vi "PicohrdlChannelSetting.vi"(5 "Unit Info":T1, 7 "Channel Settings":T2={"Ch1"={"1"=FALSE, "Ch 1"=0}, "Ch2"={"2"=FALSE, "Ch 2"=0}, "Ch3"={"3"=FALSE, "Ch 3"=0}, "Ch4"={"4"=FALSE, "Ch 4"=0}, "Ch5"={"5"=FALSE, "Ch 5"=0}, "Ch6"={"6"=FALSE, "Ch 6"=0}, "Ch7"={"7"=FALSE, "Ch 7"=0}, "Ch8"={"8"=FALSE, "Ch 8"=0}, "Ch9"={"9"=FALSE, "Ch 9"=0}, "Ch10"={"10"=FALSE, "Ch 10"=0}, "Ch11"={"11"=FALSE, "Ch 11"=0}, "Ch12"={"12"=FALSE, "Ch 12"=0}, "Ch13"={"13"=FALSE, "Ch 13"=0}, "Ch14"={"14"=FALSE, "Ch 14"=0}, "Ch15"={"15"=FALSE, "Ch 15"=0}, "Ch16"={"16"=FALSE, "Ch 16"=0}, "Ch1/Ch2"={"Single Ended"=TRUE}, "Ch3/Ch4"={"Single Ended"=TRUE}, "Ch5/Ch6"={"Single Ended"=TRUE}, "Ch7/Ch8"={"Single Ended"=TRUE}, "Ch9/Ch10"={"Single Ended"=TRUE}, "Ch11/Ch12"={"Single Ended"=TRUE}, "Ch13/Ch14"={"Single Ended"=TRUE}, "Ch15/Ch16"={"Single Ended"=TRUE}} {"Ch16"."Ch 16" items=["2500mV", "1225mV", "625mV", "313mV", "156mV", "78mV", "39mV"]; "Ch15"."Ch 15" items=["2500mV", "1225mV", "625mV", "313mV", "156mV", "78mV", "39mV"]; "Ch14"."Ch 14" items=["2500mV", "1225mV", "625mV", "313mV", "156mV", "78mV", "39mV"]; "Ch13"."Ch 13" items=["2500mV", "1225mV", "625mV", "313mV", "156mV", "78mV", "39mV"]; "Ch12"."Ch 12" items=["2500mV", "1225mV", "625mV", "313mV", "156mV", "78mV", "39mV"]; "Ch11"."Ch 11" items=["2500mV", "1225mV", "625mV", "313mV", "156mV", "78mV", "39mV"]; "Ch10"."Ch 10" items=["2500mV", "1225mV", "625mV", "313mV", "156mV", "78mV", "39mV"]; "Ch9"."Ch 9" items=["2500mV", "1225mV", "625mV", "313mV", "156mV", "78mV", "39mV"]; "Ch8"."Ch 8" items=["2500mV", "1225mV", "625mV", "313mV", "156mV", "78mV", "39mV"]; "Ch7"."Ch 7" items=["2500mV", "1225mV", "625mV", "313mV", "156mV", "78mV", "39mV"]; "Ch6"."Ch 6" items=["2500mV", "1225mV", "625mV", "313mV", "156mV", "78mV", "39mV"]; "Ch5"."Ch 5" items=["2500mV", "1225mV", "625mV", "313mV", "156mV", "78mV", "39mV"]; "Ch4"."Ch 4" items=["2500mV", "1225mV", "625mV", "313mV", "156mV", "78mV", "39mV"]; "Ch3"."Ch 3" items=["2500mV", "1225mV", "625mV", "313mV", "156mV", "78mV", "39mV"]; "Ch2"."Ch 2" items=["2500mV", "1225mV", "625mV", "313mV", "156mV", "78mV", "39mV"]; "Ch1"."Ch 1" items=["2500mV", "1225mV", "625mV", "313mV", "156mV", "78mV", "39mV"]}, 8 "error in (no error)":errorcluster, 11 "Handle In":i16=16384) -> (0 "error out":errorcluster, 1 "noOfChannels":i16=12, 2 "Channel Enable Array":i32[](array[numeric]), 3 "Handle out":i16=16384)   [LabVIEW 2010]
doc: "Calls HRDLSetAnalogInChannel() to setup channels and HRDLGetNumberOfEnabledChannels()"
uses:
  PicoHRDL.dll
  channels.ctl
panel:
  # "Diff."
  # "Diff."
  # "Diff."
  # "Diff."
  # "Diff."
  # "Diff."
  # "Diff."
  # "Diff."
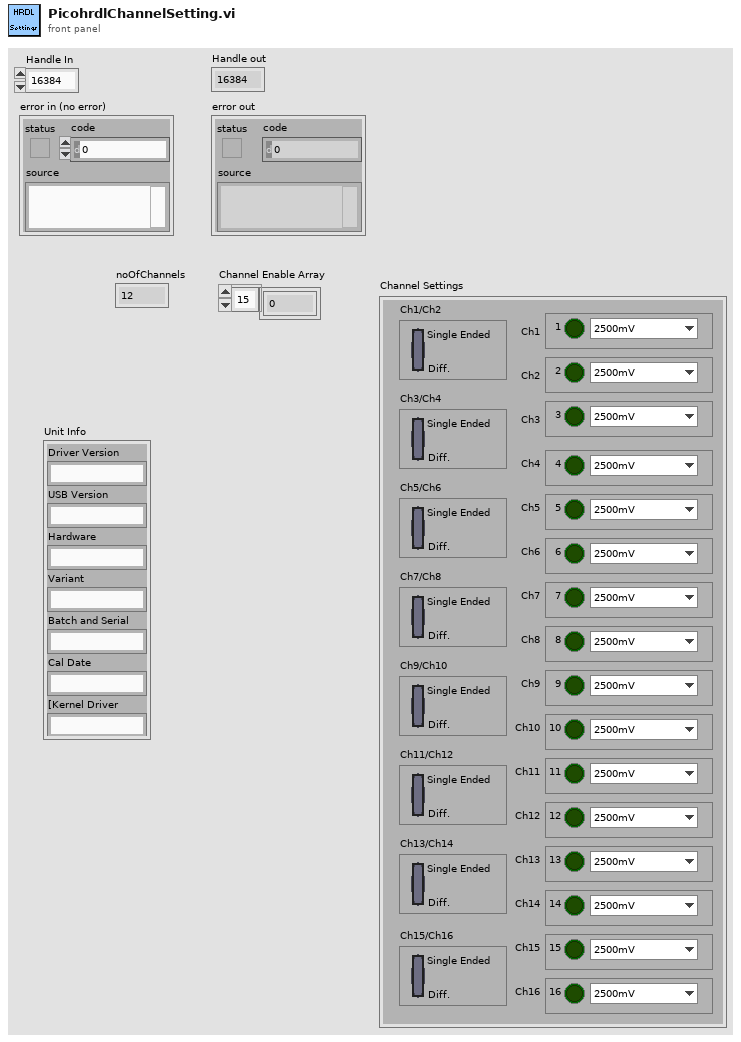
[diagram p1: front panel]
types:
  T1 = cluster{"Driver Version":string, "USB Version":string, "Hardware":string, "Variant":string, "Batch and Serial":string, "Cal Date":string, "[Kernel Driver":string, "[7]":string, "[8]":string, "[9]":string, "[10]":string, "[11]":string, "[12]":string, "[13]":string, "[14]":string}
  T2 = typedef "channels.ctl" = cluster{"Ch1":cluster{"1":bool, "Ch 1":i16}, "Ch2":cluster{"2":bool, "Ch 2":i16}, "Ch3":cluster{"3":bool, "Ch 3":i16}, "Ch4":cluster{"4":bool, "Ch 4":i16}, "Ch5":cluster{"5":bool, "Ch 5":i16}, "Ch6":cluster{"6":bool, "Ch 6":i16}, "Ch7":cluster{"7":bool, "Ch 7":i16}, "Ch8":cluster{"8":bool, "Ch 8":i16}, "Ch9":cluster{"9":bool, "Ch 9":i16}, "Ch10":cluster{"10":bool, "Ch 10":i16}, "Ch11":cluster{"11":bool, "Ch 11":i16}, "Ch12":cluster{"12":bool, "Ch 12":i16}, "Ch13":cluster{"13":bool, "Ch 13":i16}, "Ch14":cluster{"14":bool, "Ch 14":i16}, "Ch15":cluster{"15":bool, "Ch 15":i16}, "Ch16":cluster{"16":bool, "Ch 16":i16}, "Ch1/Ch2":cluster{"Single Ended":bool}, "Ch3/Ch4":cluster{"Single Ended":bool}, "Ch5/Ch6":cluster{"Single Ended":bool}, "Ch7/Ch8":cluster{"Single Ended":bool}, "Ch9/Ch10":cluster{"Single Ended":bool}, "Ch11/Ch12":cluster{"Single Ended":bool}, "Ch13/Ch14":cluster{"Single Ended":bool}, "Ch15/Ch16":cluster{"Single Ended":bool}}
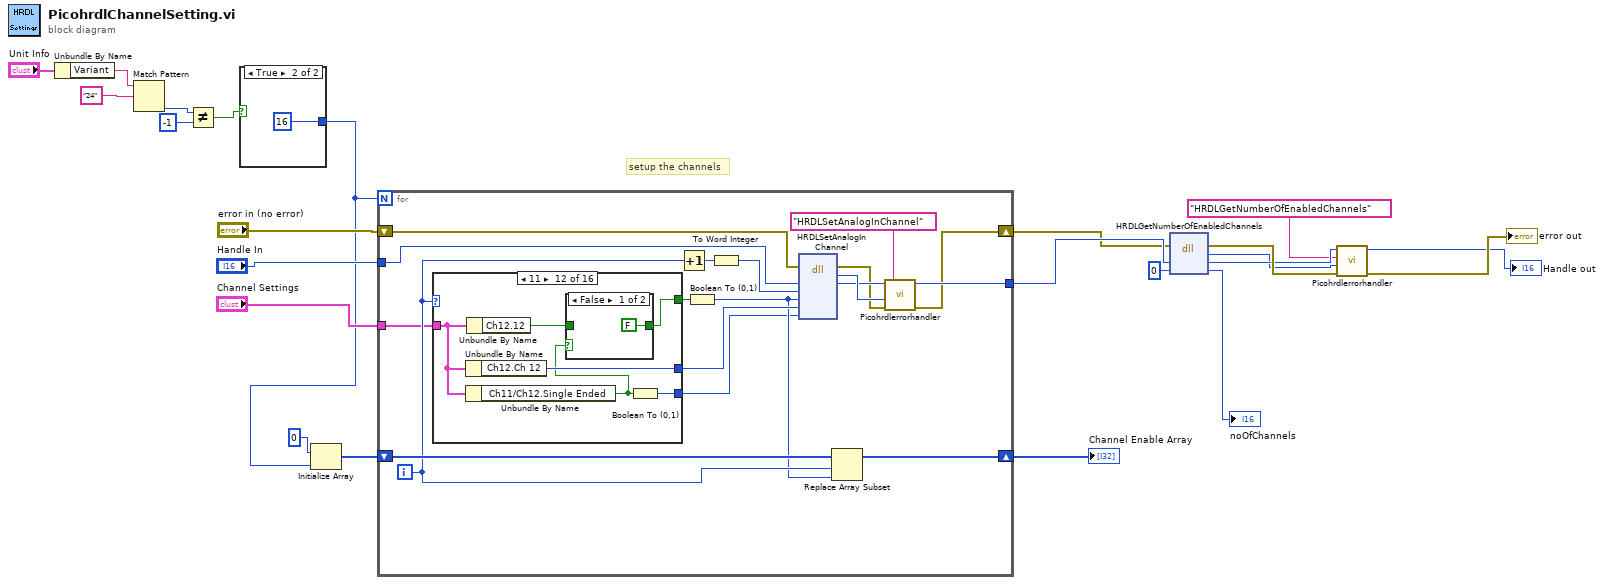
[diagram p0: block diagram]
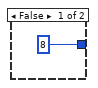
[diagram p2: hidden frame]
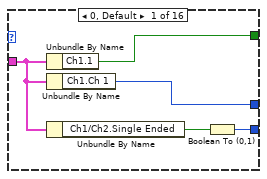
[diagram p3: hidden frame]
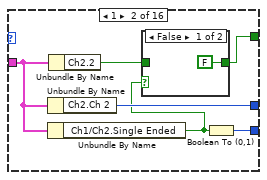
[diagram p4: hidden frame]
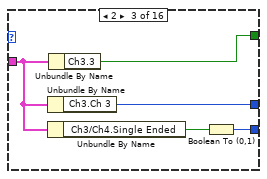
[diagram p6: hidden frame]
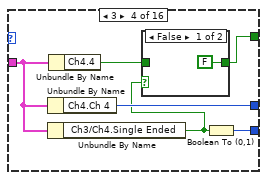
[diagram p7: hidden frame]
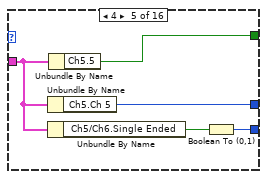
[diagram p9: hidden frame]
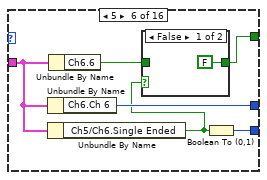
[diagram p10: hidden frame]
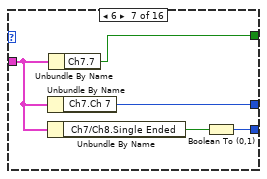
[diagram p12: hidden frame]
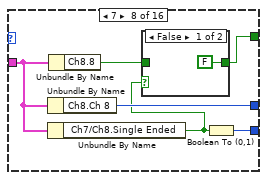
[diagram p13: hidden frame]
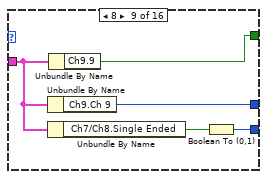
[diagram p15: hidden frame]
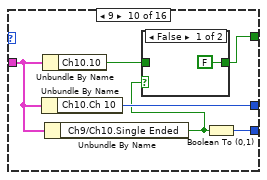
[diagram p16: hidden frame]
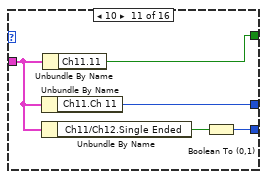
[diagram p18: hidden frame]
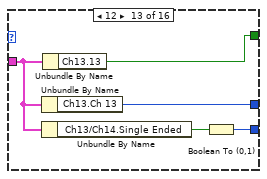
[diagram p20: hidden frame]
diagram:
  # "setup the channels"
  n1 = Unbundle By Name("Unit Info") -> ("Variant"=w6:string)
  n2 = Match Pattern(string=w6, regular expression="24") -> (offset past match=w4:i32)  [unwired: 1 in, 3 out]
  n3 = Not Equal?(x=w4, y=-1) -> (x != y?=w2:bool)
  n4 = case shown="True" w2 {
    tunnel: [8 16] -> w1
    frame False {
    }
    frame True {
    }
  }
  n5 = Initialize Array(0 ("element"), w1) -> (w20:i32[])
  n6 = for {
    N: w1 -> [_]
    shift-right: [w42] -> w22
    shift-left: w20 -> [w43]
    tunnel: "Handle In" -> [w40]
    tunnel: [w37] -> w16
    shift-right: [w26] -> w15
    shift-left: "error in (no error)" -> [w32]
    tunnel: "Channel Settings" -> [w31]
    i -> [w41]
    n7 = case shown="11" w41 {
      tunnel: [w47 w54 w61 w67 w74 w80 w87 w93 w100 w106 w113 w119 w126 w132 w139 w145] -> w39
      tunnel: [w48 w49 w57 w62 w70 w75 w83 w88 w96 w101 w109 w114 w122 w127 w135 w140] -> w38
      tunnel: w31 -> [w46 w52 w59 w65 w72 w78 w85 w91 w98 w104 w111 w117 w124 w130 w137 w143]
      tunnel: [w44 w53 w60 w66 w73 w79 w86 w92 w99 w105 w112 w118 w125 w131 w138 w144] -> w28
      frame 0, Default {
        n8 = Unbundle By Name(w46) -> ("Ch1.1"=w48:bool)
        n9 = Unbundle By Name(w46) -> ("Ch1.Ch 1"=w47:i16)
        n10 = Unbundle By Name(w46) -> ("Ch1/Ch2.Single Ended"=w45:bool)
        n11 = Boolean To (0,1)(Boolean=w45) -> (0, 1=w44:i16)
      }
      frame 1 {
        n12 = Unbundle By Name(w52) -> ("Ch2.Ch 2"=w54:i16)
        n13 = Unbundle By Name(w52) -> ("Ch1/Ch2.Single Ended"=w51:bool)
        n14 = Unbundle By Name(w52) -> ("Ch2.2"=w50:bool)
        n15 = case shown="False" w51 {
          tunnel: [FALSE ("2") w56] -> w49
          tunnel: w50 -> [_ w56]
          frame False {
          }
          frame True {
          }
        }
        n16 = Boolean To (0,1)(Boolean=w51) -> (0, 1=w53:i16)
      }
      frame 2 {
        n17 = Unbundle By Name(w59) -> ("Ch3.Ch 3"=w61:i16)
        n18 = Unbundle By Name(w59) -> ("Ch3/Ch4.Single Ended"=w58:bool)
        n19 = Unbundle By Name(w59) -> ("Ch3.3"=w57:bool)
        n20 = Boolean To (0,1)(Boolean=w58) -> (0, 1=w60:i16)
      }
      frame 3 {
        n21 = Unbundle By Name(w65) -> ("Ch4.Ch 4"=w67:i16)
        n22 = Unbundle By Name(w65) -> ("Ch3/Ch4.Single Ended"=w64:bool)
        n23 = Unbundle By Name(w65) -> ("Ch4.4"=w63:bool)
        n24 = case shown="False" w64 {
          tunnel: [FALSE ("2") w69] -> w62
          tunnel: w63 -> [_ w69]
          frame False {
          }
          frame True {
          }
        }
        n25 = Boolean To (0,1)(Boolean=w64) -> (0, 1=w66:i16)
      }
      frame 4 {
        n26 = Unbundle By Name(w72) -> ("Ch5.Ch 5"=w74:i16)
        n27 = Unbundle By Name(w72) -> ("Ch5/Ch6.Single Ended"=w71:bool)
        n28 = Unbundle By Name(w72) -> ("Ch5.5"=w70:bool)
        n29 = Boolean To (0,1)(Boolean=w71) -> (0, 1=w73:i16)
      }
      frame 5 {
        n30 = Unbundle By Name(w78) -> ("Ch6.Ch 6"=w80:i16)
        n31 = Unbundle By Name(w78) -> ("Ch5/Ch6.Single Ended"=w77:bool)
        n32 = Unbundle By Name(w78) -> ("Ch6.6"=w76:bool)
        n33 = case shown="False" w77 {
          tunnel: [FALSE ("2") w82] -> w75
          tunnel: w76 -> [_ w82]
          frame False {
          }
          frame True {
          }
        }
        n34 = Boolean To (0,1)(Boolean=w77) -> (0, 1=w79:i16)
      }
      frame 6 {
        n35 = Unbundle By Name(w85) -> ("Ch7.Ch 7"=w87:i16)
        n36 = Unbundle By Name(w85) -> ("Ch7/Ch8.Single Ended"=w84:bool)
        n37 = Unbundle By Name(w85) -> ("Ch7.7"=w83:bool)
        n38 = Boolean To (0,1)(Boolean=w84) -> (0, 1=w86:i16)
      }
      frame 7 {
        n39 = Unbundle By Name(w91) -> ("Ch8.Ch 8"=w93:i16)
        n40 = Unbundle By Name(w91) -> ("Ch7/Ch8.Single Ended"=w90:bool)
        n41 = Unbundle By Name(w91) -> ("Ch8.8"=w89:bool)
        n42 = case shown="False" w90 {
          tunnel: [FALSE ("2") w95] -> w88
          tunnel: w89 -> [_ w95]
          frame False {
          }
          frame True {
          }
        }
        n43 = Boolean To (0,1)(Boolean=w90) -> (0, 1=w92:i16)
      }
      frame 8 {
        n44 = Unbundle By Name(w98) -> ("Ch9.Ch 9"=w100:i16)
        n45 = Unbundle By Name(w98) -> ("Ch7/Ch8.Single Ended"=w97:bool)
        n46 = Unbundle By Name(w98) -> ("Ch9.9"=w96:bool)
        n47 = Boolean To (0,1)(Boolean=w97) -> (0, 1=w99:i16)
      }
      frame 9 {
        n48 = Unbundle By Name(w104) -> ("Ch10.Ch 10"=w106:i16)
        n49 = Unbundle By Name(w104) -> ("Ch10.10"=w102:bool)
        n50 = Unbundle By Name(w104) -> ("Ch9/Ch10.Single Ended"=w103:bool)
        n51 = case shown="False" w103 {
          tunnel: [FALSE ("2") w108] -> w101
          tunnel: w102 -> [_ w108]
          frame False {
          }
          frame True {
          }
        }
        n52 = Boolean To (0,1)(Boolean=w103) -> (0, 1=w105:i16)
      }
      frame 10 {
        n53 = Unbundle By Name(w111) -> ("Ch11.Ch 11"=w113:i16)
        n54 = Unbundle By Name(w111) -> ("Ch11/Ch12.Single Ended"=w110:bool)
        n55 = Unbundle By Name(w111) -> ("Ch11.11"=w109:bool)
        n56 = Boolean To (0,1)(Boolean=w110) -> (0, 1=w112:i16)
      }
      frame 11 {
        n57 = Unbundle By Name(w117) -> ("Ch12.Ch 12"=w119:i16)
        n58 = Unbundle By Name(w117) -> ("Ch11/Ch12.Single Ended"=w116:bool)
        n59 = Unbundle By Name(w117) -> ("Ch12.12"=w115:bool)
        n60 = case shown="False" w116 {
          tunnel: [FALSE ("2") w121] -> w114
          tunnel: w115 -> [_ w121]
          frame False {
          }
          frame True {
          }
        }
        n61 = Boolean To (0,1)(Boolean=w116) -> (0, 1=w118:i16)
      }
      frame 12 {
        n62 = Unbundle By Name(w124) -> ("Ch13.Ch 13"=w126:i16)
        n63 = Unbundle By Name(w124) -> ("Ch13/Ch14.Single Ended"=w123:bool)
        n64 = Unbundle By Name(w124) -> ("Ch13.13"=w122:bool)
        n65 = Boolean To (0,1)(Boolean=w123) -> (0, 1=w125:i16)
      }
      frame 13 {
        n66 = Unbundle By Name(w130) -> ("Ch14.Ch 14"=w132:i16)
        n67 = Unbundle By Name(w130) -> ("Ch13/Ch14.Single Ended"=w129:bool)
        n68 = Unbundle By Name(w130) -> ("Ch14.14"=w128:bool)
        n69 = case shown="False" w129 {
          tunnel: [FALSE ("2") w134] -> w127
          tunnel: w128 -> [_ w134]
          frame False {
          }
          frame True {
          }
        }
        n70 = Boolean To (0,1)(Boolean=w129) -> (0, 1=w131:i16)
      }
      frame 14 {
        n71 = Unbundle By Name(w137) -> ("Ch15.Ch 15"=w139:i16)
        n72 = Unbundle By Name(w137) -> ("Ch15/Ch16.Single Ended"=w136:bool)
        n73 = Unbundle By Name(w137) -> ("Ch15.15"=w135:bool)
        n74 = Boolean To (0,1)(Boolean=w136) -> (0, 1=w138:i16)
      }
      frame 15 {
        n75 = Unbundle By Name(w143) -> ("Ch16.Ch 16"=w145:i16)
        n76 = Unbundle By Name(w143) -> ("Ch15/Ch16.Single Ended"=w142:bool)
        n77 = Unbundle By Name(w143) -> ("Ch16.16"=w141:bool)
        n78 = case shown="True" w142 {
          tunnel: [FALSE ("2") w147] -> w140
          tunnel: w141 -> [_ w147]
          frame False {
          }
          frame True {
          }
        }
        n79 = Boolean To (0,1)(Boolean=w142) -> (0, 1=w144:i16)
      }
    }
    n80 = Increment(x=w41) -> (x+1=w30:i32)
    n81 = Boolean To (0,1)(Boolean=w38) -> (0, 1=w34:i16)
    n82 = To Word Integer(number=w30) -> (16bit integer=w29:i16)
    n83 = dll-call lib="PicoHRDL.dll" fn="HRDLSetAnalogInChannel"(error in=w32, "handle"=w40, "channel"=w29, "enabled"=w34, "range"=w39, "singleEnded"=w28) -> (error out=w27:errorcluster, "return type"=w36:i16, "handle"=w35:i16)  [unwired: 6 in, 1 out]
    n84 = Replace Array Subset(array=w43, new element=w34, index=w41) -> (w42:i32[])
    n85 = call "Picohrdlerrorhandler.vi"("Handle in"=w35, "API function"="HRDLSetAnalogInChannel", "Return"=w36, "error in (no error)"=w27) -> ("Handle out"=w37:i16, "error out"=w26:errorcluster)  [unwired: 5 in]
  }
  "Channel Enable Array" <- w22
  n86 = dll-call lib="PicoHRDL.dll" fn="HRDLGetNumberOfEnabledChannels"(error in=w15, "handle"=w16, "nEnabledChannels"=i16 0) -> (error out=w14:errorcluster, "return type"=w10:i16, "handle"=w11:i16, "nEnabledChannels"=→"noOfChannels":i16)  [unwired: 2 in, 1 out]
  n87 = call "Picohrdlerrorhandler.vi"("Handle in"=w11, "API function"="HRDLGetNumberOfEnabledChannels", "Return"=w10, "error in (no error)"=w14) -> ("Handle out"=→"Handle out":i16, "error out"=→"error out":errorcluster)  [unwired: 5 in]
